vi "Publish Data.vi"(7 "Message Priority (Normal)":T1, 9 "Data":refnum<class "Data.lvclass">, 10 "Actor in":refnum<class "Actor.lvclass">, 11 "Custom Multi Instrument Msg":refnum<class "Custom Multi Instrument Msg.lvclass">) -> (0 "error out":errorcluster, 2 "Actor out":refnum<class "Actor.lvclass">)   [LabVIEW 2020, in "Instrument Handler.lvlib" / "Custom Multi Instrument Msg.lvclass"]
doc: "This Vi handles the publishing of the Data from the Response Msg.\n\nThis implementation publishes with the parent method if Combined Publish is TRUE. If not it will publish each data component piece by piece."
uses:
  Custom Multi Instrument Msg.lvclass
  PPL/HDH.Data.Generic.lvlibp/Data.lvclass
  PPL/HDH.Actor Framework.Core.Actor.lvlibp/1abvi3w/vi.lib/ActorFramework/Actor/Actor.lvclass
  PPL/HDH.Actor Framework.Core.Actor.lvlibp/1abvi3w/vi.lib/ActorFramework/Message Enqueuer/Message Priority.ctl
  Custom Multi Instrument Msg.lvclass/Custom Multi Instrument Msg.ctl
  Data/Multi Instrument Data/Multi Instrument Data.lvclass
  Messages/Multi Instrument Msg/Multi Instrument Msg.lvclass
  PPL/HDH.Actor Framework.Core.Publisher.lvlibp/Messages/Timed Msg/Data/Multi Data/Multi Data.lvclass
  C:/Current projects/WS/PPL/HDH.Actor Framework.Core.Publisher.lvlibp/Messages/Timed Msg/Data/Multi Data/Multi Data.lvclass
  PPL/HDH.Actor Framework.Core.Actor.lvlibp/1abvi3w/vi.lib/ActorFramework/Message Enqueuer/Message Enqueuer.lvclass
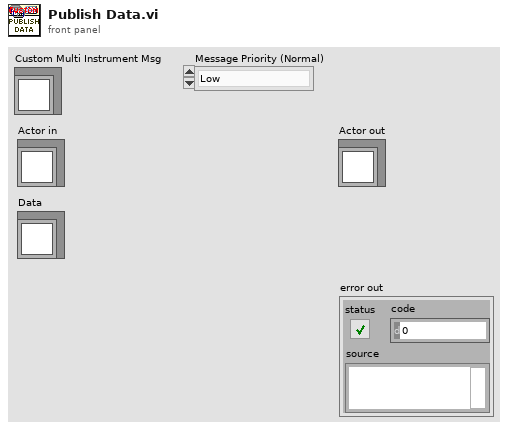
[diagram p1: front panel]
types:
  T1 = typedef "HDH.Actor Framework.Core.Actor.lvlibp/Message Enqueuer.lvclass/Message Priority.ctl" = enum16{"Low", "Normal", "High"}
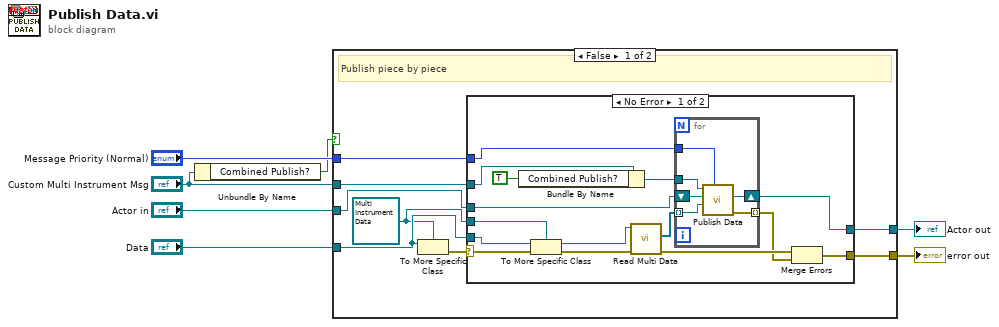
[diagram p0: block diagram]
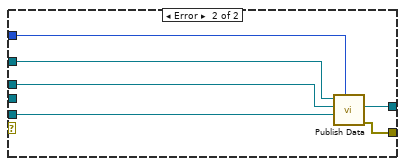
[diagram p2: hidden frame]
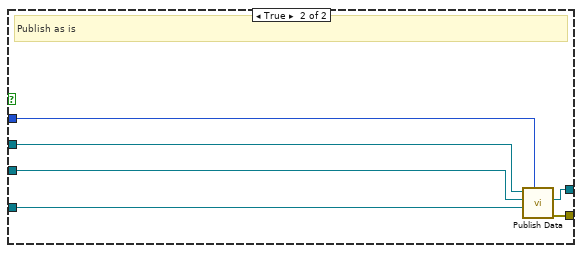
[diagram p3: hidden frame]
diagram:
  n1 = Unbundle By Name("Custom Multi Instrument Msg") -> ("Combined Publish?"=w1:bool)
  n2 = case shown="False" w1 {
    tunnel: [w10 w48] -> w7
    tunnel: [w11 w47] -> w6
    tunnel: "Message Priority (Normal)" -> [w9 w46]
    tunnel: "Data" -> [w14 w45]
    tunnel: "Actor in" -> [w12 w44]
    tunnel: "Custom Multi Instrument Msg" -> [w13 w43]
    frame False {
      w8 = refnum<class "Multi Instrument Data.lvclass"> refnum ("Instrument Handler.lvlib:Multi Instrument Data.lvclass")
      # "Publish piece by piece"
      n3 = To More Specific Class(target class=w8, reference=w14) -> (error out=w15:errorcluster)  [unwired: 1 in, 1 out]
      n4 = case shown="No Error" w15 {
        selector: w15 -> [w30 _]
        tunnel: w14 -> [w29 w37]
        tunnel: w13 -> [w25 w42]
        tunnel: w12 -> [w21 w41]
        tunnel: [w17 w40] -> w11
        tunnel: [w18 w39] -> w10
        tunnel: w9 -> [w16 w38]
        tunnel: w8 -> [w28 _]
        frame No Error {
          n5 = Bundle By Name(cluster=w25, "Combined Publish?"=TRUE) -> (w23:refnum<class "Custom Multi Instrument Msg.lvclass">)
          n6 = To More Specific Class(target class=w28, reference=w29, error in=w30) -> (specific class reference=w27:refnum<class "Multi Instrument Data.lvclass">, error out=w26:errorcluster)
          n7 = call "Read Multi Data.vi"("error in (no error)"=w26, "Multi Data in"=w27) -> ("error out"=w20:errorcluster, "Data Array"=w22:refnum<class "Data.lvclass">[])  [unwired: 5 in, 3 out]
          n8 = for {
            tunnel: w23 -> [w36]
            tunnel: w22 -> [w35] mode=indexing
            shift-right: [w33] -> w17
            shift-left: w21 -> [w34]
            tunnel: [w32] -> w19 mode=indexing
            tunnel: w16 -> [w31]
            n9 = call-parent "Publish Data.vi"("Message Priority (Normal)"=w31, "Data"=w35, "Actor in"=w34, "Response Msg"=w36) -> ("error out"=w32:errorcluster, "Actor out"=w33:refnum<class "Actor.lvclass">)  [unwired: 6 in]
          }
          n10 = Merge Errors(w20, w19) -> (w18:errorcluster)
        }
        frame Error {
          n11 = call-parent "Publish Data.vi"("Message Priority (Normal)"=w38, "Data"=w37, "Actor in"=w41, "Response Msg"=w42) -> ("error out"=w39:errorcluster, "Actor out"=w40:refnum<class "Actor.lvclass">)  [unwired: 6 in]
        }
      }
    }
    frame True {
      # "Publish as is"
      n12 = call-parent "Publish Data.vi"("Message Priority (Normal)"=w46, "Data"=w45, "Actor in"=w44, "Response Msg"=w43) -> ("error out"=w48:errorcluster, "Actor out"=w47:refnum<class "Actor.lvclass">)  [unwired: 6 in]
    }
  }
  "Actor out" <- w6
  "error out" <- w7
